vi "myRIO_BRig_RT__Case_Exp_State_initTrial_LC_ENL1__v2.vi"(6 "input_dataTrial":u16[][](array[numeric]), 7 "input_spout":enum16{"Left", "Right"}(ring), 9 "input_dataBlock":u16[][](array[numeric]), 10 "input_dataLC":u16[](array[numeric]), 11 "input_dataCurrent":u16[](array[numeric])) -> (2 "output_LC__ENL1":bool, 3 "output_LC_led__ENL1":bool, 4 "output_dataTrial":u16[][](array[numeric]), 5 "output_dataCurrent":u16[](array[numeric]))   [LabVIEW 2014]
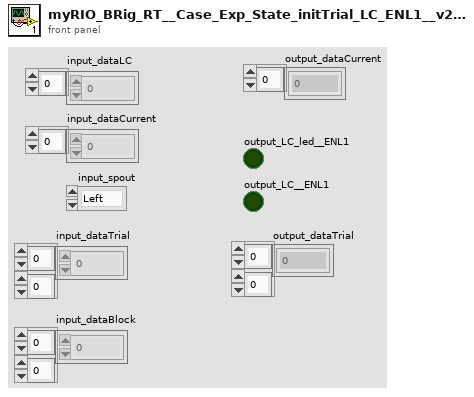
[diagram p1: front panel]
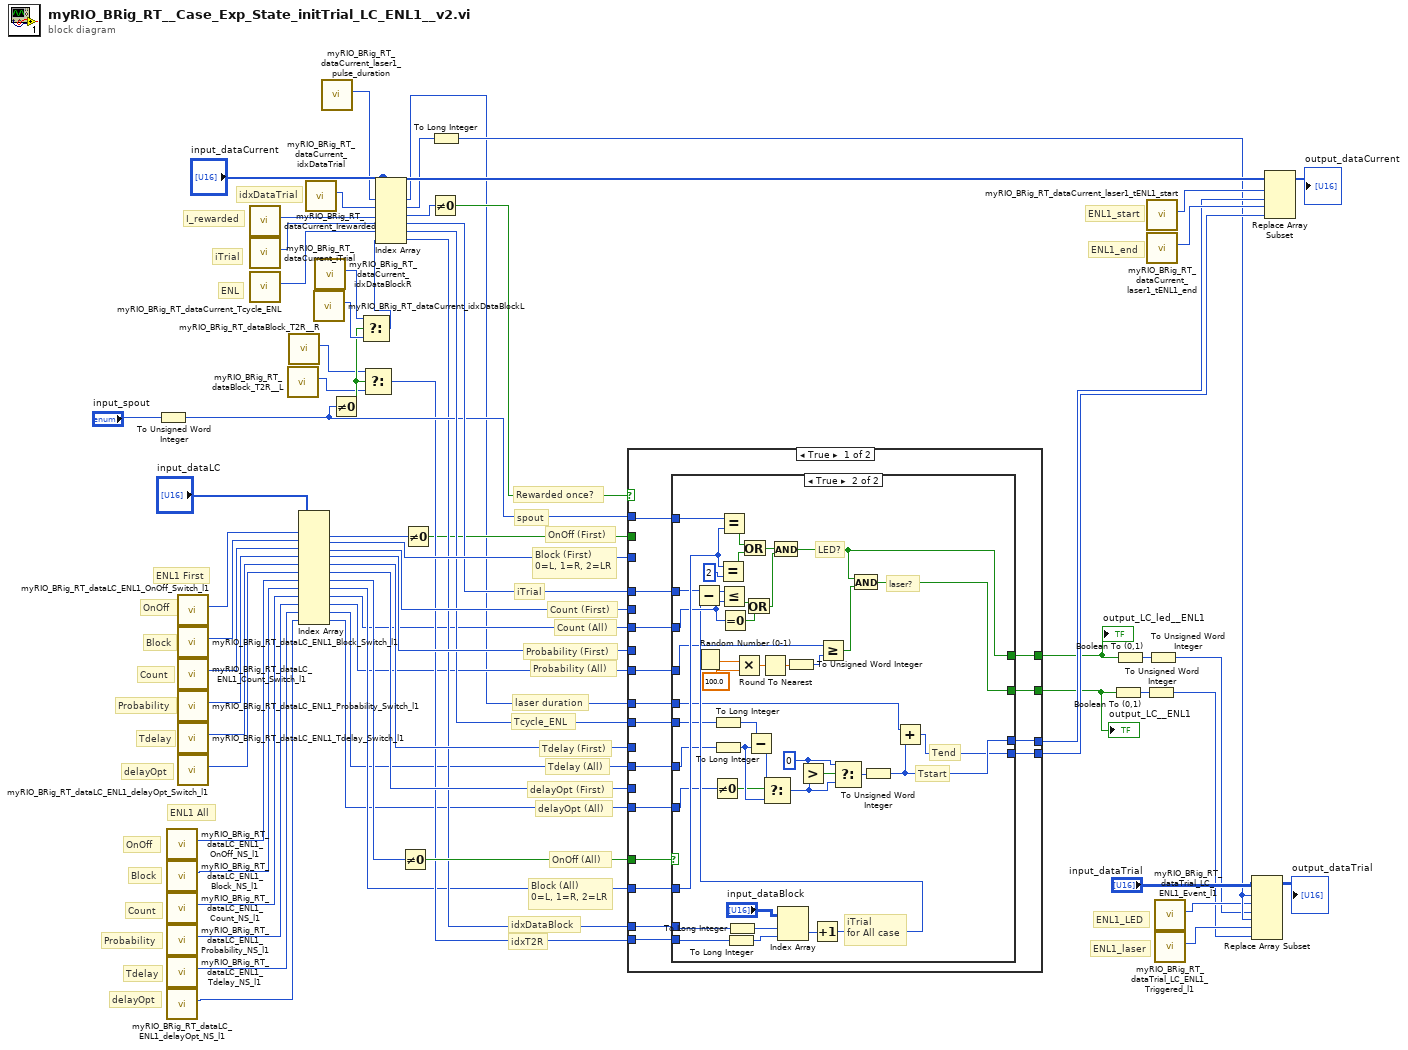
[diagram p0: block diagram]
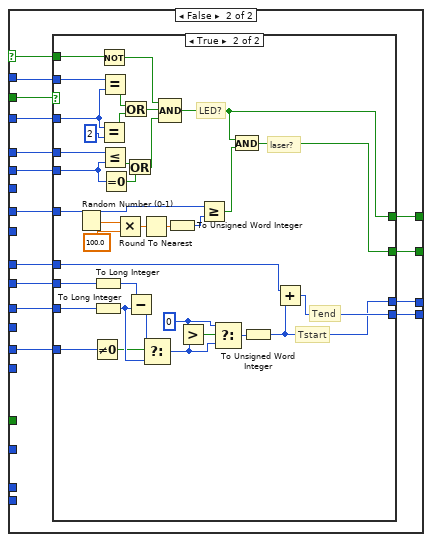
[diagram p3: hidden frame]
diagram:
  # "delayOpt (All)"
  # "Tdelay (All)"
  # "Probability (All)"
  # "Count (All)"
  # "Block (All)\n0=L, 1=R, 2=LR"
  # "idxT2R"
  # "idxDataBlock"
  # "OnOff (All)"
  # "delayOpt"
  # "Count"
  # "Tdelay"
  # "Probability"
  # "OnOff"
  # "Block"
  # "ENL1 All"
  # "Tdelay (First)"
  # "delayOpt (First)"
  # "Tcycle_ENL"
  # "laser duration"
  # "Probability (First)"
  # "Count (First)"
  # "iTrial"
  # "Block (First)\n0=L, 1=R, 2=LR"
  # "spout"
  # "Rewarded once?"
  # "OnOff (First)"
  # "iTrial"
  # "ENL1_LED"
  # "ENL1_laser"
  # "idxDataTrial"
  # "ENL1_end"
  # "ENL1_start"
  # "delayOpt"
  # "ENL"
  # "Tdelay"
  # "I_rewarded"
  # "ENL1 First"
  # "Probability"
  # "Count"
  # "Block"
  # "OnOff"
  n1 = To Unsigned Word Integer(number="input_spout") -> (unsigned 16bit integer=w24:u16)
  n2 = call "myRIO_BRig_RT_dataLC_ENL1_OnOff_NS_l1.vi"() -> ("output_ENL1_OnOff_NS_l1"=w10:i32)  [unwired: 11 in]
  n3 = call "myRIO_BRig_RT_dataLC_ENL1_Block_NS_l1.vi"() -> ("output_ENL1_All_Block"=w9:i32)  [unwired: 11 in]
  n4 = call "myRIO_BRig_RT_dataLC_ENL1_Count_NS_l1.vi"() -> ("output_ENL1_Count_NS_l1"=w8:i32)  [unwired: 11 in]
  n5 = call "myRIO_BRig_RT_dataLC_ENL1_Probability_NS_l1.vi"() -> ("output_ENL1_Probability_NS_l1"=w7:i32)  [unwired: 11 in]
  n6 = call "myRIO_BRig_RT_dataLC_ENL1_Tdelay_NS_l1.vi"() -> ("output_ENL1_Tdelay_NS_l1"=w6:i32)  [unwired: 11 in]
  n7 = call "myRIO_BRig_RT_dataLC_ENL1_delayOpt_NS_l1.vi"() -> ("output_ENL1_delayOpt_NS_l1"=w5:i32)  [unwired: 11 in]
  n8 = call "myRIO_BRig_RT_dataLC_ENL1_OnOff_Switch_l1.vi"() -> ("output_ENL1_OnOff_Switch_l1"=w64:i32)  [unwired: 11 in]
  n9 = call "myRIO_BRig_RT_dataLC_ENL1_Block_Switch_l1.vi"() -> ("output_ENL1_Block_Switch_l1"=w63:i32)  [unwired: 11 in]
  n10 = call "myRIO_BRig_RT_dataLC_ENL1_Count_Switch_l1.vi"() -> ("output_ENL1_Count_Switch_l1"=w62:i32)  [unwired: 11 in]
  n11 = call "myRIO_BRig_RT_dataLC_ENL1_Probability_Switch_l1.vi"() -> ("output_ENL1_Probability_Switch_l1"=w61:i32)  [unwired: 11 in]
  n12 = call "myRIO_BRig_RT_dataLC_ENL1_Tdelay_Switch_l1.vi"() -> ("output_ENL1_Tdelay_Switch_l1"=w53:i32)  [unwired: 11 in]
  n13 = call "myRIO_BRig_RT_dataLC_ENL1_delayOpt_Switch_l1.vi"() -> ("output_ENL1_delayOpt_Switch_l1"=w51:i32)  [unwired: 11 in]
  n14 = call "myRIO_BRig_RT_dataCurrent_Irewarded.vi"() -> ("output_I_rewarded"=w54:i32)  [unwired: 11 in]
  n15 = call "myRIO_BRig_RT_dataCurrent_iTrial.vi"() -> ("output_iTrial"=w28:i32)  [unwired: 11 in]
  n16 = call "myRIO_BRig_RT_dataCurrent_Tcycle_ENL.vi"() -> ("output_ENL"=w30:i32)  [unwired: 11 in]
  n17 = call "myRIO_BRig_RT_dataBlock_T2R__L.vi"() -> ("output_T2R__L"=w18:i32)  [unwired: 11 in]
  n18 = call "myRIO_BRig_RT_dataBlock_T2R__R.vi"() -> ("output_T2R__R"=w19:i32)  [unwired: 11 in]
  n19 = Index Array(array="input_dataLC", index #1=w64, index #2=w63, index #3=w62, index #4=w61, index #5=w53, index #6=w51, index #7=w10, index #8=w9, index #9=w8, index #10=w7, index #11=w6, index #12=w5) -> (element #1=w60:u16, element #2=w57:u16, element #3=w58:u16, element #4=w59:u16, element #5=w52:u16, element #6=w50:u16, element #7=w26:u16, element #8=w15:u16, element #9=w14:u16, element #10=w13:u16, element #11=w12:u16, element #12=w11:u16)
  n20 = call "myRIO_BRig_RT_dataCurrent_idxDataTrial.vi"() -> ("output_idxDataTrial"=w37:i32)  [unwired: 11 in]
  n21 = call "myRIO_BRig_RT_dataCurrent_idxDataBlockL.vi"() -> ("output_idxDataBlock__L"=w23:i32)  [unwired: 11 in]
  n22 = call "myRIO_BRig_RT_dataCurrent_idxDataBlockR.vi"() -> ("output_idxDataBlock__R"=w22:i32)  [unwired: 11 in]
  n23 = call "myRIO_BRig_RT_dataCurrent_laser1_pulse_duration.vi"() -> ("output_laser1_pulse_duration"=w2:i32)  [unwired: 11 in]
  n24 = Not Equal To 0?(x=w24) -> (x != 0?=w20:bool)
  n25 = Select(t=w22, s=w20, f=w23) -> (s? t:f=w21:i32)
  n26 = Select(t=w19, s=w20, f=w18) -> (s? t:f=w16:i32)
  n27 = Index Array(array="input_dataCurrent", index #1=w2, index #2=w37, index #3=w54, index #4=w28, index #5=w30, index #6=w21) -> (element #1=w1:u16, element #2=w36:u16, element #3=w55:u16, element #4=w27:u16, element #5=w29:u16, element #6=w17:u16)
  n28 = Not Equal To 0?(x=w26) -> (x != 0?=w25:bool)
  n29 = Not Equal To 0?(x=w60) -> (x != 0?=w3:bool)
  n30 = Not Equal To 0?(x=w55) -> (x != 0?=w4:bool)
  n31 = To Long Integer(number=w36) -> (32bit integer=w35:i32)
  n32 = case shown="True" w4 {
    selector: w4 -> [_ w125]
    tunnel: w57 -> [_ w137]
    tunnel: w58 -> [_ w128]
    tunnel: w59 -> [_ w135]
    tunnel: [w78 w133] -> w40
    tunnel: [w79 w134] -> w42
    tunnel: w24 -> [w81 w138]
    tunnel: w52 -> [_ w130]
    tunnel: w50 -> [_ w131]
    tunnel: w29 -> [w74 w127]
    tunnel: w1 -> [w75 w126]
    tunnel: [w76 w129] -> w45
    tunnel: [w77 w132] -> w44
    tunnel: w27 -> [w80 w136]
    tunnel: w25 -> [w66 _]
    tunnel: w16 -> [w73 _]
    tunnel: w17 -> [w72 _]
    tunnel: w15 -> [w71 _]
    tunnel: w14 -> [w70 _]
    tunnel: w13 -> [w69 _]
    tunnel: w12 -> [w68 _]
    tunnel: w11 -> [w67 _]
    tunnel: w3 -> [_ w124]
    frame True {
      n33 = case shown="True" w66 {
        tunnel: w81 -> [_ w122]
        tunnel: w80 -> [_ w101]
        tunnel: [_ w96] -> w79
        tunnel: [_ w113] -> w78
        tunnel: [_ w85] -> w77
        tunnel: [_ w86] -> w76
        tunnel: w75 -> [_ w87]
        tunnel: w74 -> [_ w84]
        tunnel: w73 -> [_ w107]
        tunnel: w72 -> [_ w109]
        tunnel: w71 -> [_ w104]
        tunnel: w70 -> [_ w103]
        tunnel: w69 -> [_ w99]
        tunnel: w68 -> [_ w83]
        tunnel: w67 -> [_ w82]
        frame False {
        }
        frame True {
          w93 = 0 ("x")
          # "Tstart"
          # "Tend"
          # "iTrial\nfor All case"
          # "laser?"
          # "LED?"
          n34 = Random Number (0-1)() -> (number: 0 to 1=w119:dbl)
          n35 = Not Equal To 0?(x=w82) -> (x != 0?=w90:bool)
          n36 = To Long Integer(number=w84) -> (32bit integer=w88:i32)
          n37 = To Long Integer(number=w83) -> (32bit integer=w91:i32)
          n38 = Equal?(x=w104, y=u16 2) -> (x = y?=w120:bool)
          n39 = Equal?(x=w122, y=w104) -> (x = y?=w121:bool)
          n40 = Equal To 0?(x=w103) -> (x = 0?=w111:bool)
          n41 = To Long Integer(number=w107) -> (32bit integer=w106:i32)
          n42 = To Long Integer(number=w109) -> (32bit integer=w108:i32)
          n43 = Multiply(x=w119, y=100.0) -> (x*y=w118:dbl)
          n44 = Or(x=w121, y=w120) -> (x .or. y?=w98:bool)
          n45 = Subtract(x=w88, y=w91) -> (x-y=w89:i32)
          n46 = Round To Nearest(number=w118) -> (nearest integer value=w117:dbl)
          n47 = Select(t=w89, s=w90, f=w91) -> (s? t:f=w94:i32)
          n48 = Index Array(array="input_dataBlock", index (row)=w108, index (col)=w106) -> (element=w105:u16)
          n49 = To Unsigned Word Integer(number=w117) -> (unsigned 16bit integer=w115:u16)
          n50 = Greater?(x=w93, y=w94) -> (0:w92:bool)
          n51 = Increment(x=w105) -> (x+1=w102:u16)
          n52 = Subtract(x=w101, y=w102) -> (x-y=w100:u16)
          n53 = Less Or Equal?(x=w100, y=w103) -> (x <= y?=w112:bool)
          n54 = Or(x=w112, y=w111) -> (x .or. y?=w97:bool)
          n55 = And(x=w98, y=w97) -> (x .and. y?=w96:bool)
          n56 = Greater Or Equal?(x=w99, y=w115) -> (x >= y?=w114:bool)
          n57 = Select(t=w93, s=w92, f=w94) -> (s? t:f=w95:i32)
          n58 = And(x=w96, y=w114) -> (x .and. y?=w113:bool)
          n59 = To Unsigned Word Integer(number=w95) -> (unsigned 16bit integer=w86:u16)
          n60 = Add(x=w87, y=w86) -> (x+y=w85:u16)
        }
      }
    }
    frame False {
      n61 = case shown="True" w124 {
        tunnel: w138 -> [_ w173]
        tunnel: w137 -> [_ w172]
        tunnel: w136 -> [_ w171]
        tunnel: w135 -> [_ w164]
        tunnel: [_ w159] -> w134
        tunnel: [_ w158] -> w133
        tunnel: [_ w140] -> w132
        tunnel: w131 -> [_ w144]
        tunnel: w130 -> [_ w142]
        tunnel: [_ w139] -> w129
        tunnel: w128 -> [_ w157]
        tunnel: w127 -> [_ w143]
        tunnel: w126 -> [_ w141]
        tunnel: w125 -> [_ w153]
        frame False {
        }
        frame True {
          w150 = 0 ("x")
          # "Tstart"
          # "Tend"
          # "laser?"
          # "LED?"
          n62 = Random Number (0-1)() -> (number: 0 to 1=w168:dbl)
          n63 = Not Equal To 0?(x=w144) -> (x != 0?=w147:bool)
          n64 = To Long Integer(number=w143) -> (32bit integer=w145:i32)
          n65 = To Long Integer(number=w142) -> (32bit integer=w148:i32)
          n66 = Not(x=w153) -> (.not. x?=w162:bool)
          n67 = Equal?(x=w172, y=u16 2) -> (x = y?=w169:bool)
          n68 = Equal?(x=w173, y=w172) -> (x = y?=w170:bool)
          n69 = Less Or Equal?(x=w171, y=w157) -> (x <= y?=w156:bool)
          n70 = Equal To 0?(x=w157) -> (x = 0?=w155:bool)
          n71 = Multiply(x=w168, y=100.0) -> (x*y=w167:dbl)
          n72 = Or(x=w170, y=w169) -> (x .or. y?=w161:bool)
          n73 = Or(x=w156, y=w155) -> (x .or. y?=w154:bool)
          n74 = Subtract(x=w145, y=w148) -> (x-y=w146:i32)
          n75 = Round To Nearest(number=w167) -> (nearest integer value=w166:dbl)
          n76 = Select(t=w146, s=w147, f=w148) -> (s? t:f=w151:i32)
          n77 = Compound Arithmetic op=AND(w162, w161, w154) -> (w159:bool)
          n78 = To Unsigned Word Integer(number=w166) -> (unsigned 16bit integer=w163:u16)
          n79 = Greater?(x=w150, y=w151) -> (0:w149:bool)
          n80 = Greater Or Equal?(x=w164, y=w163) -> (x >= y?=w160:bool)
          n81 = Select(t=w150, s=w149, f=w151) -> (s? t:f=w152:i32)
          n82 = And(x=w159, y=w160) -> (x .and. y?=w158:bool)
          n83 = To Unsigned Word Integer(number=w152) -> (unsigned 16bit integer=w139:u16)
          n84 = Add(x=w141, y=w139) -> (x+y=w140:u16)
        }
      }
    }
  }
  "output_LC__ENL1" <- w40
  "output_LC_led__ENL1" <- w42
  n85 = Boolean To (0,1)(Boolean=w40) -> (0, 1=w41:i16)
  n86 = Boolean To (0,1)(Boolean=w42) -> (0, 1=w43:i16)
  n87 = To Unsigned Word Integer(number=w41) -> (unsigned 16bit integer=w31:u16)
  n88 = call "myRIO_BRig_RT_dataCurrent_laser1_tENL1_start.vi"() -> ("output_laser1_tENL1_start"=w47:i32)  [unwired: 11 in]
  n89 = call "myRIO_BRig_RT_dataCurrent_laser1_tENL1_end.vi"() -> ("output_laser1_tENL1_end"=w46:i32)  [unwired: 11 in]
  n90 = To Unsigned Word Integer(number=w43) -> (unsigned 16bit integer=w32:u16)
  n91 = call "myRIO_BRig_RT_dataTrial_LC_ENL1_Event_l1.vi"() -> ("output_LC_ENL1_Event_l1"=w34:i32)  [unwired: 11 in]
  n92 = call "myRIO_BRig_RT_dataTrial_LC_ENL1_Triggered_l1.vi"() -> ("output_LC_ENL1_Triggered_l1"=w33:i32)  [unwired: 11 in]
  n93 = Replace Array Subset(array="input_dataTrial", new element #1=w32, index (row) #1=w35, index (col) #1=w34, new element #2=w31, index (row) #2=w35, index (col) #2=w33) -> (→"output_dataTrial":u16[][])
  n94 = Replace Array Subset(array="input_dataCurrent", new element #1=w45, index #1=w47, new element #2=w44, index #2=w46) -> (→"output_dataCurrent":u16[])
